vi "LVCAM Nest Destroyed.vi"(10 "Nest Actor":refnum<class "LVCAM.lvclass">, 11 "LVCAM Nest Destroyed Msg in":refnum<class "LVCAM Nest Destroyed Msg.lvclass">) -> (0 "error out":errorcluster, 3 "LVCAM Nest Destroyed Msg out":refnum<class "LVCAM Nest Destroyed Msg.lvclass">)   [LabVIEW 2021, in "LVCAM Nest Destroyed.lvlib" / "LVCAM Nest Destroyed Msg.lvclass"]
uses:
  LVCAM Nest Destroyed Msg.lvclass
  LVCAM/LVCAM/LVCAM.lvclass
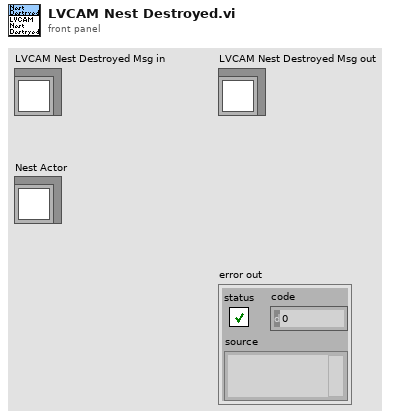
[diagram p1: front panel]
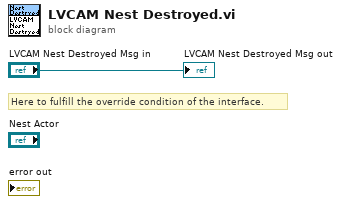
[diagram p0: block diagram]
diagram:
  # "Here to fulfill the override condition of the interface."
  "LVCAM Nest Destroyed Msg out" <- "LVCAM Nest Destroyed Msg in"
